vi "AO_mini_wavefrontShow.vi"() -> ()   [LabVIEW 2018]
uses:
  <userlib>/WaveKit.lib/Controls/StatisticsData.ctl
  <userlib>/WaveKit.lib/Controls/HasoSlopes.lvclass
  <userlib>/WaveKit.lib/Controls/WavefrontReconstructionMode.ctl
  <userlib>/WaveKit.lib/Classes/Phase/Phase.lvclass
  <userlib>/WaveKit.lib/Controls/Pupil.lvclass
panel:
  in  "Save File":bool
  in  "Filter":u8[](array[numeric])
  out "Phase values":sgl[][](graph) caption="Wavefront"
  out "Phase statistics":T1
  in  "idxType":enum16{"Wyant", "ANSI"}(ring)=enum."ANSI"
  in  "Output folder":path=path "D:/Data"
  in  "Output file name":string="zern_coeffs.txt"
  in  "Hasao slopes file":path=path "D:/Data/20211215_DMresponse/fullAnalysis_ANSI/ANSI_idx_3/0p5_slopesNet.has"
  out "Zernike Coefficients":dbl[](graph)
  out "error out":errorcluster
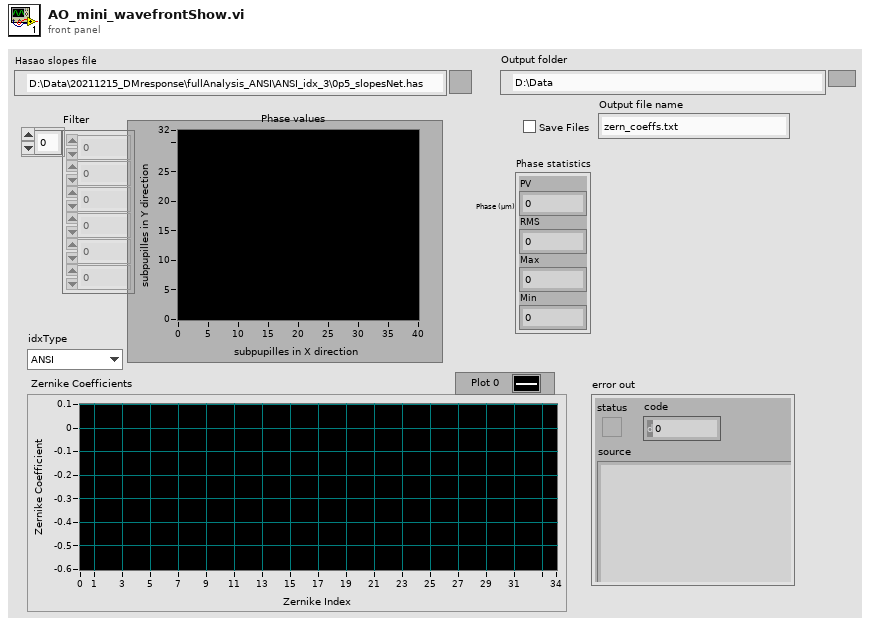
[diagram p1: front panel]
types:
  T1 = typedef "StatisticsData.ctl" = cluster{"PV":sgl, "RMS":dbl, "Max":sgl, "Min":sgl}
  T2 = typedef "WavefrontReconstructionMode.ctl" = enum16{"None", "Modal_Legendre", "Modal_Zernike", "Zonal", "Modal_Zonal_Zernike", "Modal_Zonal_Legendre"}
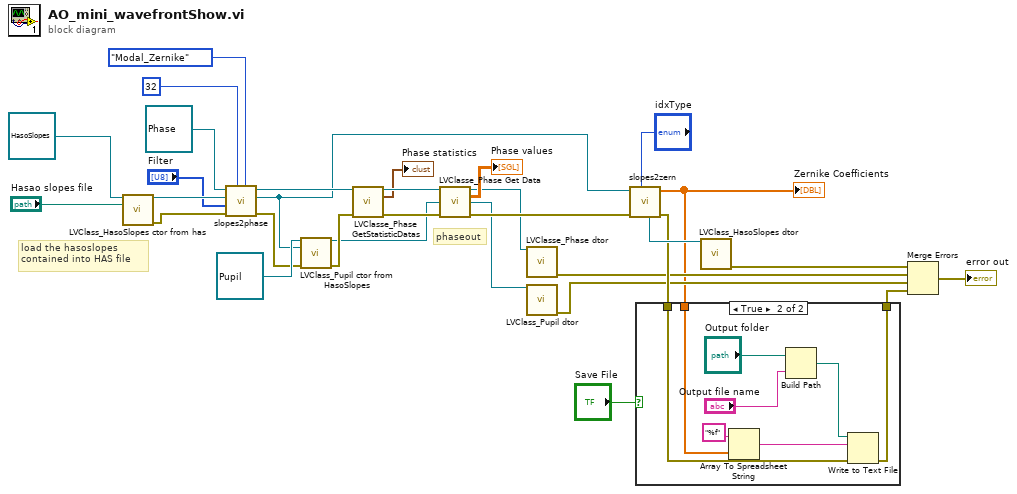
[diagram p0: block diagram]
diagram:
  # "phaseout"
  # "load the hasoslopes\ncontained into HAS file"
  n1 = call <userlib>:"LVClass_HasoSlopes ctor from has.vi"("HasoSlopes in"=refnum<class "HasoSlopes.lvclass"> refnum, ".has path"="Hasao slopes file") -> ("HasoSlopes out"=w19:refnum<class "HasoSlopes.lvclass">, "error out"=w17:errorcluster)  [unwired: 12 in]
  n2 = call "slopes2phase.vi"("TypePhase"=WavefrontReconstructionMode."Modal_Zernike", "Number of coefficients"=u8 32, "error in (no error)"=w17, "Filter"="Filter", "HasoSlopes in"=w19, "Phase in"=refnum<class "Phase.lvclass"> refnum) -> ("error out"=w16:errorcluster, "HasoSlopes out"=w11:refnum<class "HasoSlopes.lvclass">, "Phase out"=w15:refnum<class "Phase.lvclass">)  [unwired: 3 in]
  n3 = call <userlib>:"LVClass_Pupil ctor from HasoSlopes.vi"("Pupil in"=refnum<class "Pupil.lvclass"> refnum, "HasoSlopes.lvclass"=w11, "error in (no error)"=w16) -> ("Pupil out"=w13:refnum<class "Pupil.lvclass">, "error out"=w14:errorcluster)  [unwired: 11 in]
  n4 = call <userlib>:"LVClasse_Phase GetStatisticDatas.vi"("Phase in"=w15, "error in (no error)"=w14) -> ("Phase out"=w24:refnum<class "Phase.lvclass">, "StatisticsData"=→"Phase statistics":T1, "error out"=w22:errorcluster)  [unwired: 11 in]
  n5 = call <userlib>:"LVClasse_Phase Get Data.vi"("Phase in"=w24, "Pupil"=w13, "error in (no error)"=w22) -> ("Phase out"=w9:refnum<class "Phase.lvclass">, "data"=→"Phase values":sgl[][], "Pupil (dup)"=w10:refnum<class "Pupil.lvclass">, "error out"=w12:errorcluster)  [unwired: 9 in]
  n6 = call <userlib>:"LVClasse_Phase dtor.vi"("Phase in"=w9) -> ("error out"=w5:errorcluster)  [unwired: 13 in, 1 out]
  n7 = call <userlib>:"LVClass_Pupil dtor.vi"("Pupil in"=w10) -> ("error out"=w4:errorcluster)  [unwired: 13 in, 1 out]
  n8 = call "slopes2zern.vi"("HasoSlopes in"=w11, "error in (no error)"=w12, "idxType"="idxType") -> ("HasoSlopes out"=w29:refnum<class "HasoSlopes.lvclass">, "Zernike Coefficients"=w1:dbl[], "error out"=w8:errorcluster)  [unwired: 3 in, 2 out]
  "Zernike Coefficients" <- w1
  n9 = case shown="True" "Save File" {
    tunnel: w1 -> [_ w35]
    tunnel: w8 -> [w32 w34]
    tunnel: [w32 w33] -> w3
    frame False {
    }
    frame True {
      n10 = Array To Spreadsheet String(array=w35, 3:"%f") -> (spreadsheet string=w39:string)  [unwired: 1 in]
      n11 = Build Path(base path="Output folder", name or relative path="Output file name") -> (appended path=w36:path)
      n12 = Write to Text File(file (use dialog)=w36, text=w39, error in=w34) -> (error out=w33:errorcluster)  [unwired: 1 in, 2 out]
    }
  }
  n13 = call <userlib>:"LVClass_HasoSlopes dtor.vi"("HasoSlopes in"=w29) -> ("error out"=w6:errorcluster)  [unwired: 13 in, 1 out]
  n14 = Merge Errors(w6, w5, w4, w3) -> (→"error out":errorcluster)
